vi "ROI group-Groups control menu handler.vi"(9 "ItemTag":string, 11 "ROI groups window notifier":refnum<notifier>) -> ()   [LabVIEW 2013]
uses:
  ROI grouping window/Typedefs/ROI grp-process states enum.ctl
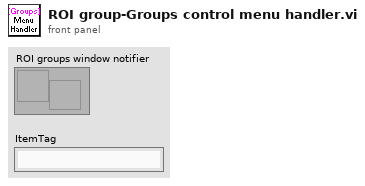
[diagram p1: front panel]
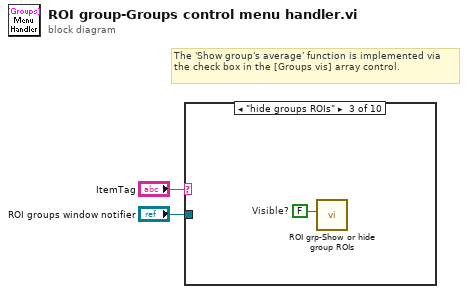
[diagram p0: block diagram]
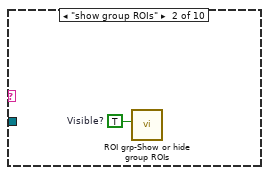
[diagram p3: hidden frame]
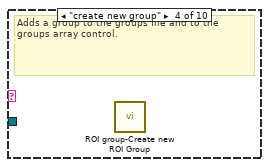
[diagram p4: hidden frame]
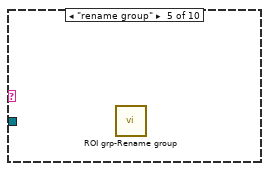
[diagram p5: hidden frame]
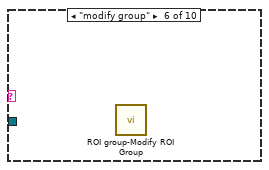
[diagram p6: hidden frame]
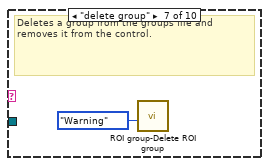
[diagram p7: hidden frame]
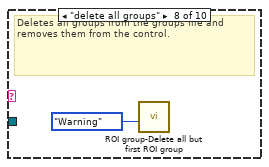
[diagram p8: hidden frame]
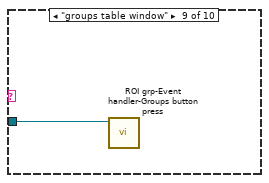
[diagram p9: hidden frame]
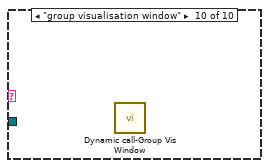
[diagram p10: hidden frame]
diagram:
  # "The 'Show group's average' function is implemented via the check box in the [Groups vis] array control."
  n1 = case shown="\"hide groups ROIs\"" "ItemTag" {
    tunnel: "ROI groups window notifier" -> [_ _ _ _ _ _ _ _ w7 _]
    frame Default {
    }
    frame "show group ROIs" {
      w3 = TRUE  # Visible?
      n2 = call "ROI grp-Show or hide group ROIs.vi"("Visible?"=w3) -> ()  [unwired: 10 in, 1 out]
    }
    frame "hide groups ROIs" {
      w4 = FALSE  # Visible?
      n3 = call "ROI grp-Show or hide group ROIs.vi"("Visible?"=w4) -> ()  [unwired: 10 in, 1 out]
    }
    frame "create new group" {
      # "Adds a group to the groups file and to the groups array control."
      n4 = call "ROI group-Create new ROI Group.vi"() -> ()  [unwired: 10 in, 2 out]
    }
    frame "rename group" {
      n5 = call "ROI grp-Rename group.vi"() -> ()  [unwired: 12 in]
    }
    frame "modify group" {
      n6 = call "ROI group-Modify ROI Group.vi"() -> ()  [unwired: 9 in, 3 out]
    }
    frame "delete group" {
      # "Deletes a group from the groups file and removes it from the control."
      n7 = call "ROI group-Delete ROI group.vi"("Dialogue message type"=enum16{"Warning", "Attention"}."Warning") -> ()  [unwired: 11 in]
    }
    frame "delete all groups" {
      # "Deletes all groups from the groups file and removes them from the control."
      n8 = call "ROI group-Delete all but first ROI group.vi"("Dialogue message type"=enum16{"Warning", "Attention"}."Warning") -> ()  [unwired: 10 in, 1 out]
    }
    frame "groups table window" {
      n9 = call "ROI grp-Event handler-Groups button press.vi"("Groups window notifier"=w7) -> ()  [unwired: 11 in]
    }
    frame "group visualisation window" {
      n10 = call "Dynamic call-Group Vis Window.vi"() -> ()  [unwired: 11 in, 1 out]
    }
  }
